vi "Simple image acquisition mono - polling.vi"() -> ()   [LabVIEW 2015]
uses:
  C:/code/Host/Installer/Scientific Camera Interfaces/LabVIEW/32_bit/Library_X86/Thorlabs.TSI.TLCameraInterfaces.dll
  code/Host/Installer/Scientific Camera Interfaces/LabVIEW/32_bit/Library_X86/Thorlabs.TSI.TLCameraInterfaces.dll
  C:/code/Host/Installer/Scientific Camera Interfaces/LabVIEW/32_bit/Library_X86/Thorlabs.TSI.TLCamera.dll
  code/Host/Installer/Scientific Camera Interfaces/LabVIEW/32_bit/Library_X86/Thorlabs.TSI.TLCamera.dll
  C:/code/Host/Installer/Scientific Camera Interfaces/LabVIEW/32_bit/Library_X86/Thorlabs.TSI.ImageDataInterfaces.dll
  code/Host/Installer/Scientific Camera Interfaces/LabVIEW/32_bit/Library_X86/Thorlabs.TSI.ImageDataInterfaces.dll
panel:
  in  "Exposure (ms)":u32=100
  out "FrameNumber":u32
  out "Intensity Graph Mono":u16[][](graph)
  in  "stop":bool
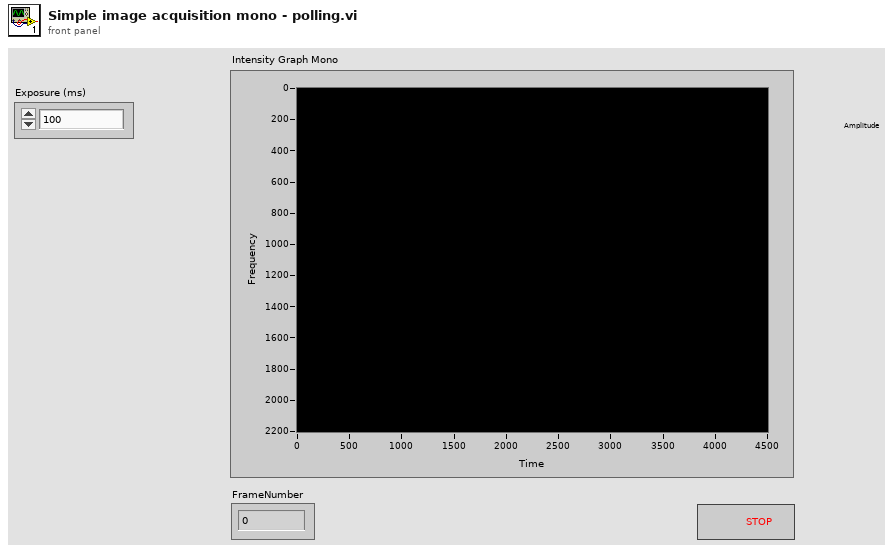
[diagram p1: front panel]
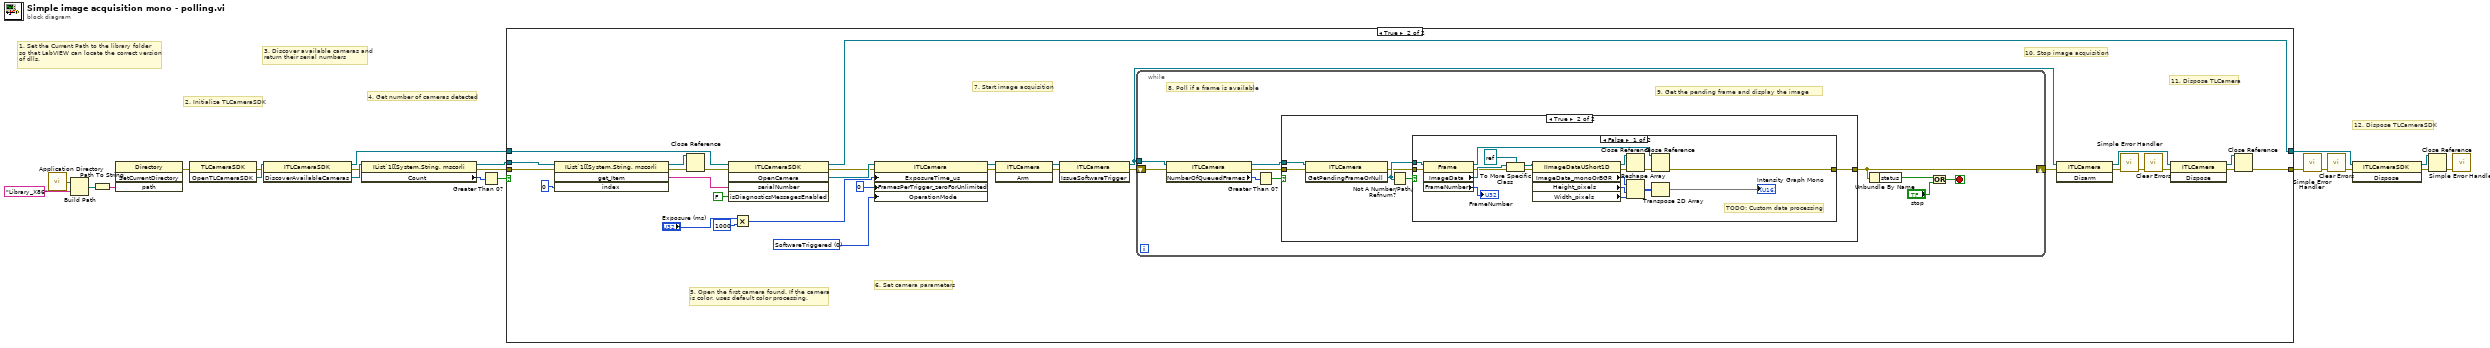
[diagram p0: block diagram]
diagram:
  # "1. Set the Current Path to the library folder\nso that LabVIEW can locate the correct version\nof dlls."
  # "12. Dispose TLCameraSDK"
  # "4. Get number of cameras detected"
  # "3. Discover available cameras and\nreturn their serial numbers"
  # "2. Initialize TLCameraSDK"
  n1 = call <vilib>:"Application Directory.vi"() -> ("Application Directory"=w8:path)
  n2 = Build Path(base path=w8, name or relative path="Library_X86") -> (appended path=w6:path)
  n3 = Path To String(path=w6) -> (string=w5:string)
  n4 = invoke class="Directory" method="SetCurrentDirectory"("path"=w5) -> (error out=w4:errorcluster)  [unwired: 3 in, 3 out]
  n5 = invoke class="TLCameraSDK" method="OpenTLCameraSDK"(error in=w4) -> (error out=w9:errorcluster, "OpenTLCameraSDK"=w10:refnum<k24>)  [unwired: 2 in, 1 out]
  n6 = invoke class="ITLCameraSDK" method="DiscoverAvailableCameras"(reference=w10, error in=w9) -> (reference out=w13:refnum<k24>, error out=w15:errorcluster, "DiscoverAvailableCameras"=w16:refnum<k24>)  [unwired: 1 in]
  n7 = property class="IList`1[[System.String, mscorli"(reference=w16, error in=w15) -> (reference out=w12:refnum<k24>, error out=w11:errorcluster, "Count"=w14:i32)
  n8 = Greater Than 0?(x=w14) -> (x > 0?=w17:bool)
  n9 = case shown="True" w17 {
    tunnel: w13 -> [w22 w54]
    tunnel: w11 -> [w23 w45]
    tunnel: [w23 w48] -> w2
    tunnel: [w22 w47] -> w21
    tunnel: w12 -> [_ w46]
    frame False {
    }
    frame True {
      w32 = 0 items=["SoftwareTriggered", "HardwareTriggered", "Bulb", "Reserved1", "Reserved2"] ("OperationMode")
      # "11. Dispose TLCamera"
      # "10. Stop image acquisition"
      # "7. Start image acquisition"
      # "6. Set camera parameters"
      # "5. Open the first camera found. If the camera\nis color, uses default color processing."
      n10 = invoke class="IList`1[[System.String, mscorli" method="get_Item"(reference=w46, error in=w45, "index"=0) -> (reference out=w44:refnum<k24>, error out=w43:errorcluster, "get_Item"=w40:string)  [unwired: 1 in, 1 out]
      n11 = Close Reference(reference=w44, error in (no error)=w43) -> (error out=w42:errorcluster)
      n12 = invoke class="ITLCameraSDK" method="OpenCamera"(reference=w54, error in=w42, "serialNumber"=w40, "isDiagnosticsMessagesEnabled"=FALSE) -> (reference out=w47:refnum<k24>, error out=w34:errorcluster, "OpenCamera"=w35:refnum<k24>)  [unwired: 1 in, 2 out]
      n13 = Multiply(x="Exposure (ms)", y=u32 1000) -> (x*y=w33:u32)
      n14 = property class="ITLCamera"(reference=w35, error in=w34, "ExposureTime_us"=w33, "FramesPerTrigger_zeroForUnlimited"=u32 0 ("FramesPerTriggerOrZeroForUnlimited"), "OperationMode"=w32) -> (reference out=w25:refnum<k24>, error out=w24:errorcluster)
      n15 = invoke class="ITLCamera" method="Arm"(reference=w25, error in=w24) -> (reference out=w39:refnum<k24>, error out=w38:errorcluster)  [unwired: 1 in, 1 out]
      n16 = invoke class="ITLCamera" method="IssueSoftwareTrigger"(reference=w39, error in=w38) -> (reference out=w37:refnum<k24>, error out=w36:errorcluster)  [unwired: 1 in, 1 out]
      n17 = while {
        tunnel: w37 -> [w64]
        shift-right: [w58] -> w29
        shift-left: w36 -> [w63]
        stop <- w55 stop-if-true
        # "9. Get the pending frame and display the image"
        # "8. Poll if a frame is available"
        n18 = property class="ITLCamera"(reference=w64, error in=w63) -> (reference out=w59:refnum<k24>, error out=w60:errorcluster, "NumberOfQueuedFrames"=w62:i32)
        n19 = Greater Than 0?(x=w62) -> (x > 0?=w61:bool)
        n20 = case shown="True" w61 {
          tunnel: w60 -> [w65 w70]
          tunnel: w59 -> [_ w71]
          tunnel: [w65 w66] -> w58
          frame False {
          }
          frame True {
            n21 = invoke class="ITLCamera" method="GetPendingFrameOrNull"(reference=w71, error in=w70) -> (error out=w67:errorcluster, "GetPendingFrameOrNull"=w68:refnum<k24>)  [unwired: 1 in, 1 out]
            n22 = Not A Number/Path/Refnum?(number/path/refnum=w68) -> (NaN/Path/Refnum?=w69:bool)
            n23 = case shown="False" w69 {
              tunnel: w68 -> [w78 _]
              tunnel: w67 -> [w88 w90]
              tunnel: [w83 w90] -> w66
              frame False {
                # "TODO: Custom data processing"
                n24 = property class="Frame"(reference=w78, error in=w88) -> (reference out=w85:refnum<k24>, error out=w75:errorcluster, "ImageData"=w76:refnum<k24>, "FrameNumber"=→"FrameNumber":u32)
                n25 = To More Specific Class(target class=refnum<k24> refnum, reference=w76, error in=w75) -> (specific class reference=w73:refnum<k24>, error out=w74:errorcluster)
                n26 = property class="IImageDataUShort1D"(reference=w73, error in=w74) -> (reference out=w86:refnum<k24>, error out=w87:errorcluster, "ImageData_monoOrBGR"=w89:u16[], "Height_pixels"=w80:i32, "Width_pixels"=w81:i32)
                n27 = Close Reference(reference=w86, error in (no error)=w87) -> (error out=w84:errorcluster)
                n28 = Reshape Array(w89, w80, w81) -> (w77:u16[][])
                n29 = Close Reference(reference=w85, error in (no error)=w84) -> (error out=w83:errorcluster)
                n30 = Transpose 2D Array(2D array=w77) -> (transposed array=→"Intensity Graph Mono":u16[][])
              }
              frame True {
              }
            }
          }
        }
        n31 = Unbundle By Name(w58) -> ("status"=w57:bool)
        n32 = Or(x=w57, y="stop") -> (x .or. y?=w55:bool)
      }
      n33 = invoke class="ITLCamera" method="Disarm"(reference=w37, error in=w29) -> (reference out=w51:refnum<k24>, error out=w28:errorcluster)  [unwired: 1 in, 1 out]
      n34 = call <vilib>:"Simple Error Handler.vi"("error in (no error)"=w28) -> ("error out"=w27:errorcluster)  [unwired: 4 in, 4 out]
      n35 = call <vilib>:"Clear Errors.vi"("error in (no error)"=w27) -> ("error out"=w26:errorcluster)  [unwired: 5 in, 1 out]
      n36 = invoke class="ITLCamera" method="Dispose"(reference=w51, error in=w26) -> (reference out=w49:refnum<k24>, error out=w50:errorcluster)  [unwired: 1 in, 1 out]
      n37 = Close Reference(reference=w49, error in (no error)=w50) -> (error out=w48:errorcluster)
    }
  }
  n38 = call <vilib>:"Simple Error Handler.vi"("error in (no error)"=w2) -> ("error out"=w3:errorcluster)  [unwired: 4 in, 4 out]
  n39 = call <vilib>:"Clear Errors.vi"("error in (no error)"=w3) -> ("error out"=w1:errorcluster)  [unwired: 5 in, 1 out]
  n40 = invoke class="ITLCameraSDK" method="Dispose"(reference=w21, error in=w1) -> (reference out=w20:refnum<k24>, error out=w19:errorcluster)  [unwired: 1 in, 1 out]
  n41 = Close Reference(reference=w20, error in (no error)=w19) -> (error out=w18:errorcluster)
  n42 = call <vilib>:"Simple Error Handler.vi"("error in (no error)"=w18) -> ()  [unwired: 4 in, 5 out]
